vi "Obtain Request Events.vi"(8 "error in":errorcluster, 10 "Create New? (F)":bool) -> (0 "error out":errorcluster, 2 "DAQ Request Events":T1)   [LabVIEW 2024, in "DAQ.lvlib"]
doc: "This VI Obtains/Creates the Requests events that will be used for other modules to communicate with the module that owns this VI. These Requests events will be accessed only via Public API methods for this module.\n\n<b>NOTE</b>: The contents of this VI are automatically generated and modified by the <b>Tools > DQMH Consortium > DQMH</b> utilities. Consider using those utilities instead of making your own modifications to this VI.\n_____\nBased on DQMH Project Template 7.0.1.1316."
uses:
  DAQ.lvlib
  Request Events--cluster.ctl
  Stop Argument--cluster.ctl
  Show Panel Argument--cluster.ctl
  Hide Panel Argument--cluster.ctl
  Get Module Execution Status Argument--cluster.ctl
  Show Diagram Argument--cluster.ctl
  Configure Acquisition Argument--cluster.ctl
  DAQ Config.ctl
  Start Acquisition Argument--cluster.ctl
  Acquire Argument--cluster.ctl
  Stop Acquisition Argument--cluster.ctl
panel:
  # "NOTE: The contents of this VI are automatically generated and modified by the Tools > DQMH Consortium > DQMH utilities. Consider using those utilities instead of making your own modifications to this VI."
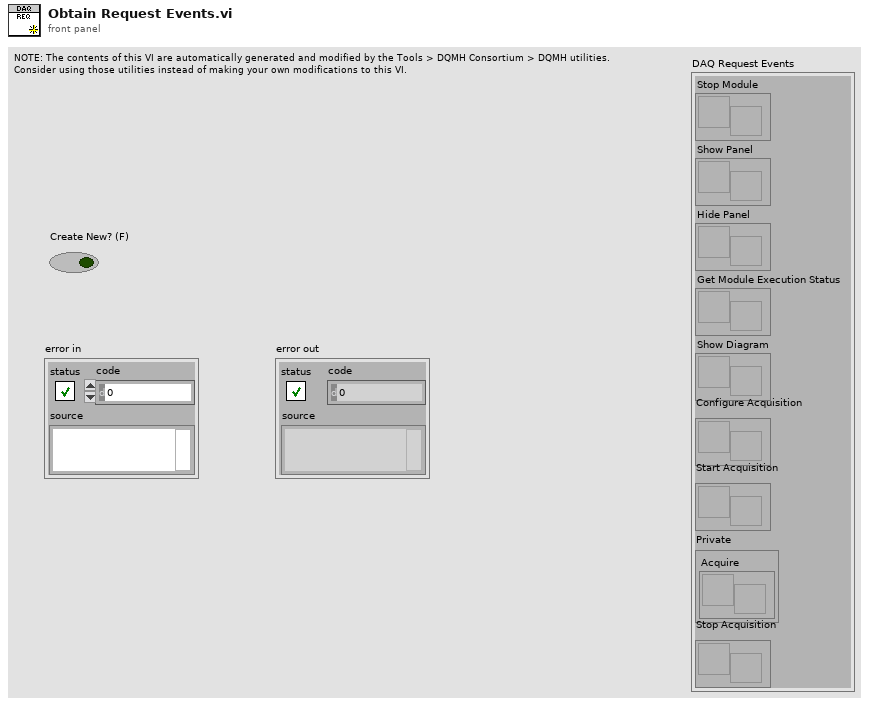
[diagram p1: front panel]
types:
  T1 = typedef "DAQ.lvlib/Request Events--cluster.ctl" = cluster{"Stop Module":refnum<user-event>, "Show Panel":refnum<user-event>, "Hide Panel":refnum<user-event>, "Get Module Execution Status":refnum<user-event>, "Show Diagram":refnum<user-event>, "Configure Acquisition":refnum<user-event>, "Start Acquisition":refnum<user-event>, "Private":cluster{"Acquire":refnum<user-event>}, "Stop Acquisition":refnum<user-event>}
  T2 = typedef "DAQ.lvlib/Stop Acquisition Argument--cluster.ctl" = cluster{"Boolean":bool}
  T3 = typedef "DAQ.lvlib/Acquire Argument--cluster.ctl" = cluster{"Boolean":bool}
  T4 = typedef "DAQ.lvlib/Start Acquisition Argument--cluster.ctl" = cluster{"Boolean":bool}
  T5 = typedef "DAQ.lvlib/Configure Acquisition Argument--cluster.ctl" = cluster{"DAQ Config":T6}
  T6 = typedef "DAQ.lvlib/DAQ Config.ctl" = cluster{"DAQmx Channel":tag, "Samplerate":dbl}
  T7 = typedef "DAQ.lvlib/Hide Panel Argument--cluster.ctl" = cluster{"Hide Panel?":bool}
  T8 = typedef "DAQ.lvlib/Show Panel Argument--cluster.ctl" = cluster{"Show Panel?":bool}
  T9 = typedef "DAQ.lvlib/Show Diagram Argument--cluster.ctl" = cluster{"Debug?":bool}
  T10 = typedef "DAQ.lvlib/Get Module Execution Status Argument--cluster.ctl" = cluster{"Running?":bool}
  T11 = typedef "DAQ.lvlib/Stop Argument--cluster.ctl" = cluster{"Origin":string, "Exit via Stop Module Req?":bool, "Wait for Module to stop?":bool}
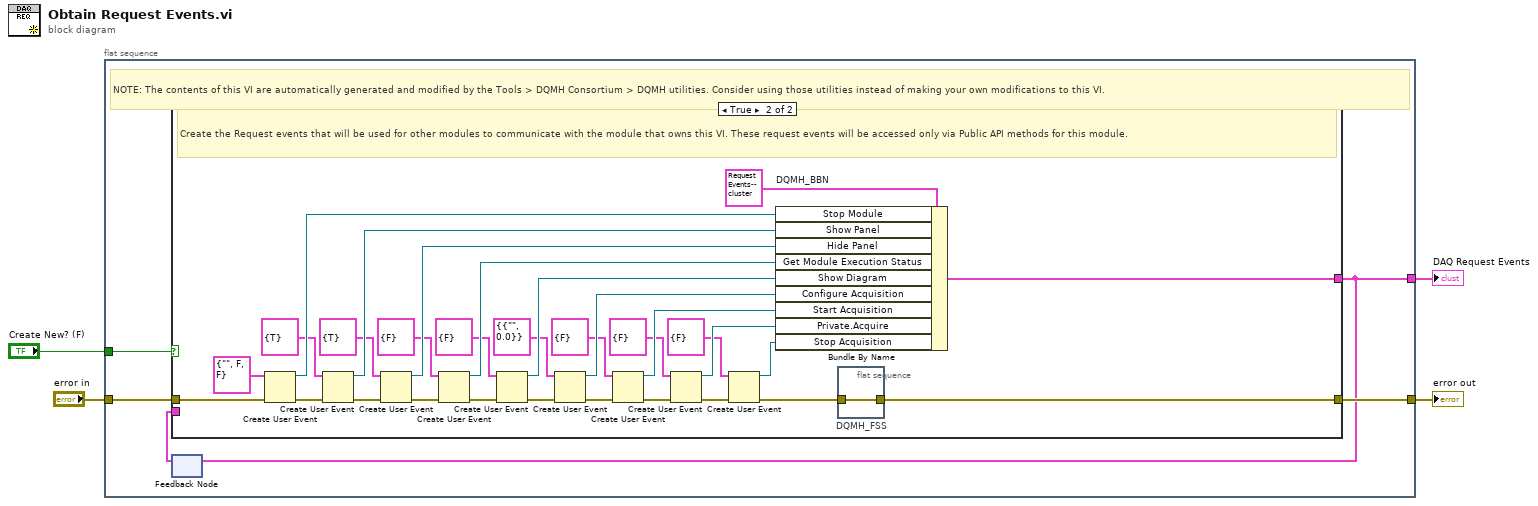
[diagram p0: block diagram]
diagram:
  n1 = flat-sequence {
    tunnel: [w9] -> w4
    tunnel: "error in" -> [w8]
    tunnel: [w6] -> w2
    tunnel: "Create New? (F)" -> [w5]
    frame #0 {
      # "NOTE: The contents of this VI are automatically generated and modified by the Tools > DQMH Consortium > DQMH utilities. Consider using those utilities instead of making your own modifications to this VI."
      n2 = feedback #1() -> (w7:T1)  [unwired: 1 in]
      n3 = case shown="True" w5 {
        tunnel: [w10 w32] -> w9
        tunnel: w8 -> [w10 w42]
        tunnel: [w11 w39] -> w6
        tunnel: w7 -> [w11 _]
        frame False {
          # "Obtain the Request events that were created in a previous call to this VI."
        }
        frame True {
          # "Create the Request events that will be used for other modules to communicate with the module that owns this VI. These request events will be accessed only via Public API methods for this module."
          n4 = Create User Event(user event datatype=T11 {"Origin"="", "Exit via Stop Module Req?"=FALSE, "Wait for Module to stop?"=FALSE} ("Stop Argument"), error in=w42) -> (user event=w40:refnum<user-event>, error out=w37:errorcluster)
          n5 = Create User Event(user event datatype=T8 {"Show Panel?"=TRUE} ("Show Panel Argument"), error in=w37) -> (user event=w36:refnum<user-event>, error out=w35:errorcluster)
          n6 = Create User Event(user event datatype=T7 {"Hide Panel?"=TRUE} ("Hide Panel Argument"), error in=w35) -> (user event=w34:refnum<user-event>, error out=w33:errorcluster)
          n7 = Create User Event(user event datatype=T10 {"Running?"=FALSE} ("Get Module Execution Status Argument"), error in=w33) -> (user event=w30:refnum<user-event>, error out=w31:errorcluster)
          n8 = Create User Event(user event datatype=T9 {"Debug?"=FALSE} ("Show Diagram Argument"), error in=w31) -> (user event=w27:refnum<user-event>, error out=w28:errorcluster)
          n9 = Create User Event(user event datatype=T5 {"DAQ Config"={"DAQmx Channel"="", "Samplerate"=0.0}} ("Configure Acquisition Argument"), error in=w28) -> (user event=w22:refnum<user-event>, error out=w23:errorcluster)
          n10 = Create User Event(user event datatype=T4 {"Boolean"=FALSE} ("Start Acquisition Argument"), error in=w23) -> (user event=w19:refnum<user-event>, error out=w20:errorcluster)
          n11 = Create User Event(user event datatype=T3 {"Boolean"=FALSE} ("Acquire Argument"), error in=w20) -> (user event=w16:refnum<user-event>, error out=w17:errorcluster)
          n12 = Create User Event(user event datatype=T2 {"Boolean"=FALSE} ("Stop Acquisition Argument"), error in=w17) -> (user event=w13:refnum<user-event>, error out=w14:errorcluster)
          n13 = Bundle By Name "DQMH_BBN"(cluster=T1 {"Stop Module"=refnum, "Show Panel"=refnum, "Hide Panel"=refnum, "Get Module Execution Status"=refnum, "Show Diagram"=refnum, "Configure Acquisition"=refnum, "Start Acquisition"=refnum, "Private"={"Acquire"=refnum}, "Stop Acquisition"=refnum} ("output cluster"), "Stop Module"=w40, "Show Panel"=w36, "Hide Panel"=w34, "Get Module Execution Status"=w30, "Show Diagram"=w27, "Configure Acquisition"=w22, "Start Acquisition"=w19, "Private.Acquire"=w16, "Stop Acquisition"=w13) -> (w39:T1)
          n14 = flat-sequence "DQMH_FSS" {
            tunnel: w14 -> [w43]
            tunnel: [w43] -> w32
            frame #0 {
            }
          }
        }
      }
      n15 = feedback-in #1(w6) -> ()
    }
  }
  "DAQ Request Events" <- w2
  "error out" <- w4
